vi "Command Get Status.vi"(8 "Password":string, 9 "Username":string, 11 "Target IP Address":string) -> (0 "error out":errorcluster, 2 "Status":string)   [LabVIEW 2020]
uses:
  Web Service/Endpoints.ctl
  <vilib>/httpClient/LabVIEWHTTPClient.lvlib
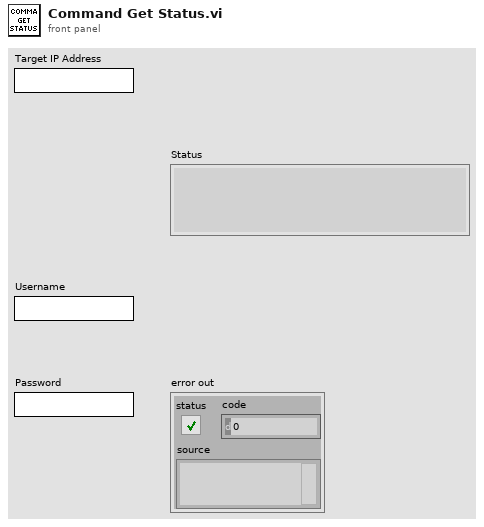
[diagram p1: front panel]
types:
  T1 = typedef "Endpoints.ctl" = string
  T2 = typedef "LabVIEWHTTPClient.lvlib/ClientHandle.ctl" = refnum<k1>
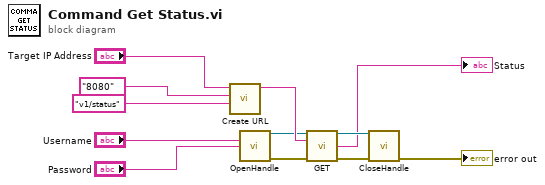
[diagram p0: block diagram]
diagram:
  n1 = call "Create URL.vi"("endpoint"=T1 "v1/status", "port"="8080", "Target IP Address"="Target IP Address") -> ("URL Out"=w11:string)  [unwired: 8 in]
  n2 = call <vilib>:"OpenHandle.vi"("username"="Username", "password"="Password") -> ("client handle out"=w3:T2, "error out"=w2:errorcluster)  [unwired: 12 in]
  n3 = call <vilib>:"GET.vi"("client handle"=w3, "url"=w11, "error in (no error)"=w2) -> ("client handle out"=w5:T2, "body"=→"Status":string, "error out"=w4:errorcluster)  [unwired: 9 in, 1 out]
  n4 = call <vilib>:"CloseHandle.vi"("client handle"=w5, "error in (no error)"=w4) -> ("error out"=→"error out":errorcluster)  [unwired: 13 in]
